vi "lab4_usrp_cp_ofdm_transceiver.vi"() -> ()   [LabVIEW 2014]
uses:
  <vilib>/addons/Modulation/Digital/General/MT Generate Bits (Galois, PN Order).vi
  <vilib>/Analysis/2dsp.llb/Inverse Complex FFT.vi
  <vilib>/Analysis/2dsp.llb/Complex FFT.vi
  <vilib>/Analysis/5stat.llb/RMS (DBL).vi
  <vilib>/addons/Modulation/Digital/Support/Common/Validators/mod_Generate Bits Validate.vi
  <vilib>/addons/Modulation/Analog/support/mod_Set Error Source.vi
  var_stop.vi
  <vilib>/addons/Modulation/Digital/Support/Common/Validators/mod_Generate Filter Coefficients Validate.vi
  <vilib>/addons/Modulation/Digital/General/subVIs/mod_Generate Filter Coefficients.vi
  <vilib>/addons/Modulation/Digital/General/subVIs/mod_Generate Bits PN Sequence.vi
  <vilib>/addons/Modulation/Digital/General/MT Generate QAM System Parameters(M).vi
  <vilib>/addons/Modulation/Digital/General/MT Apply Pulse Shaping Filter (Generic).vi
  <instrlib>/niUSRP/niUSRP Write Tx Data (CDB Cluster).vi
  <vilib>/addons/Modulation/Digital/General/MT Apply Matched Filter (Generic).vi
  <vilib>/addons/Modulation/Digital/General/MT Align to Ideal Symbols (Generic).vi
  <vilib>/addons/Modulation/Digital/General/MT Map QAM Symbols to Bits.vi
  <instrlib>/niUSRP/niUSRP Fetch Rx Data (CDB Cluster).vi
  <vilib>/addons/Modulation/niDMT.lvlib
  <vilib>/Analysis/NI_AALPro.lvlib
panel:
  out "Time domain ofdm signal":dbl[](graph)
  out "Frequency domain subcarrier magnitude":dbl[](graph)
  out "PAPR":dbl
  in  "M-QAM (16)":i32=16
  out "TX buffer":i32
  out "RX buffer":i32
  out "avg energy":dbl
  in  "TX on":bool=TRUE
  in  "power scale":dbl format="%#_13g"
  out "acc recieved bits":i32
  out "acc error bits":i32
  out "Packet number":u8
  out "Packet bytes":u32
  out "past 20 error bits":i32[](array[numeric])
  in  "min_len":i32=200
  in  "Threshold":dbl=-61.0 format="%#_13g"
  out "Accumulated BER":dbl
  out "found packet":bool
  in  "total bits (128)":i32=1600 caption="bits per packet"
  in  "message carriers":i32=120
  out "RX  constellation map":cdb[](graph)
  in  "pilot carrier":i32=32
  in  "cyclic length":i32=64
  in  "FFT size":i32=256
  in  "filter length (symbols)":i32=8
  in  "filter parameter":dbl=0.35 format="%.2f"
  in  "samples per symbol (16)":i32=4
  in  "pulse shaping filter (none)":T1(ring)=enum."Root Raised Cos"
  in  "stop":bool
  in  "number of samples":i64=20000
  out "coerced carrier frequency":dbl format="%#_6p"
  out "coerced IQ rate":dbl format="%#_6p"
  in  "Clocking and Synchronization:Reference Frequency Source":string(combo)="Internal"
  in  "RX gain":dbl format="%#_6f"
  in  "TX gain":dbl format="%#_6f"
  in  "carrier frequency":dbl=915000000.0 format="%#_6p"
  in  "IQ rate":dbl=2000000.0 format="%#_6p"
  in  "RX device names":refnum<k15>="192.168.10.3"
  in  "TX device names":refnum<k15>="192.168.10.3"
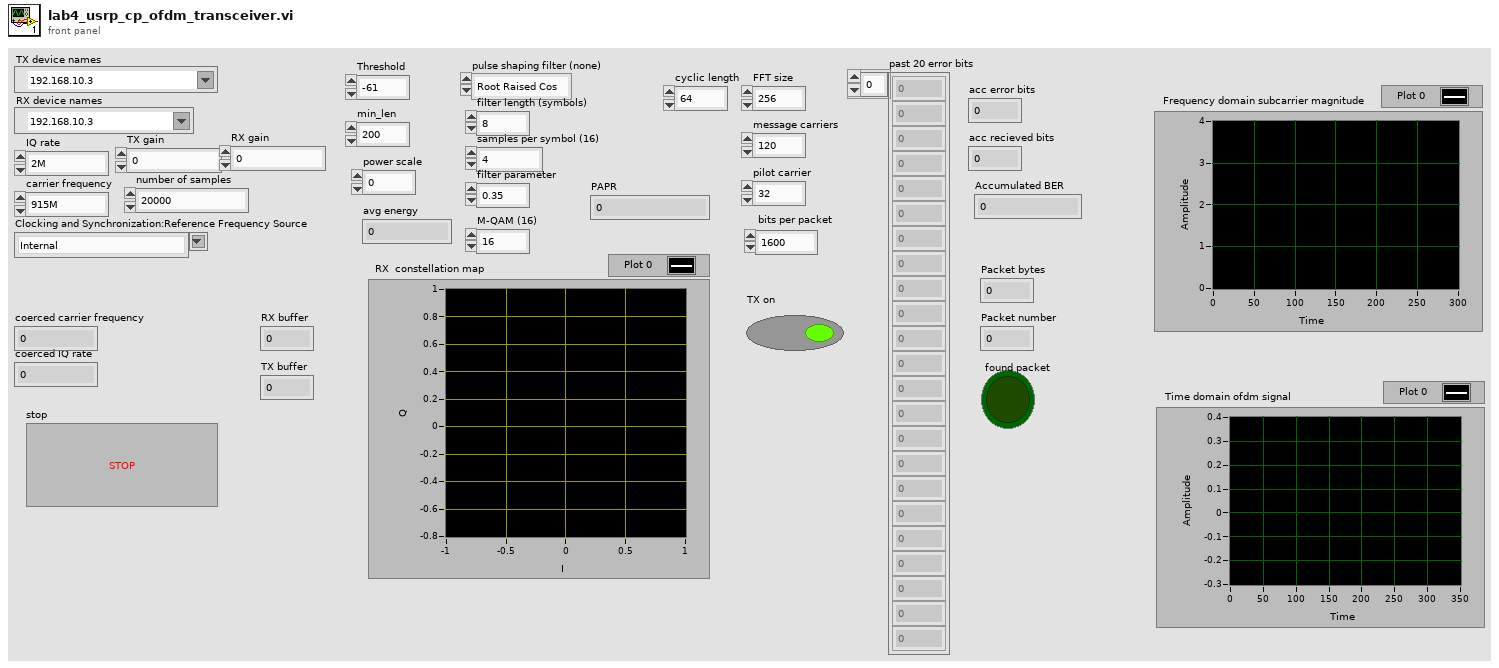
[diagram p1: front panel]
types:
  T1 = enum16{"none", "Raised Cosine", "Root Raised Cos", "Gaussian"}
  T2 = enum16{"FSK", "PSK", "QAM", "MSK", "PAM", "ASK", "CPM"}
  T3 = cluster{"samples per symbol (16)":i32, "symbol map":cdb[]}
  T4 = typedef "niAMT.lvlib/Complex Data Waveform.ctl" = cluster{"t0":dbl, "dt":dbl, "Y":cdb[]}
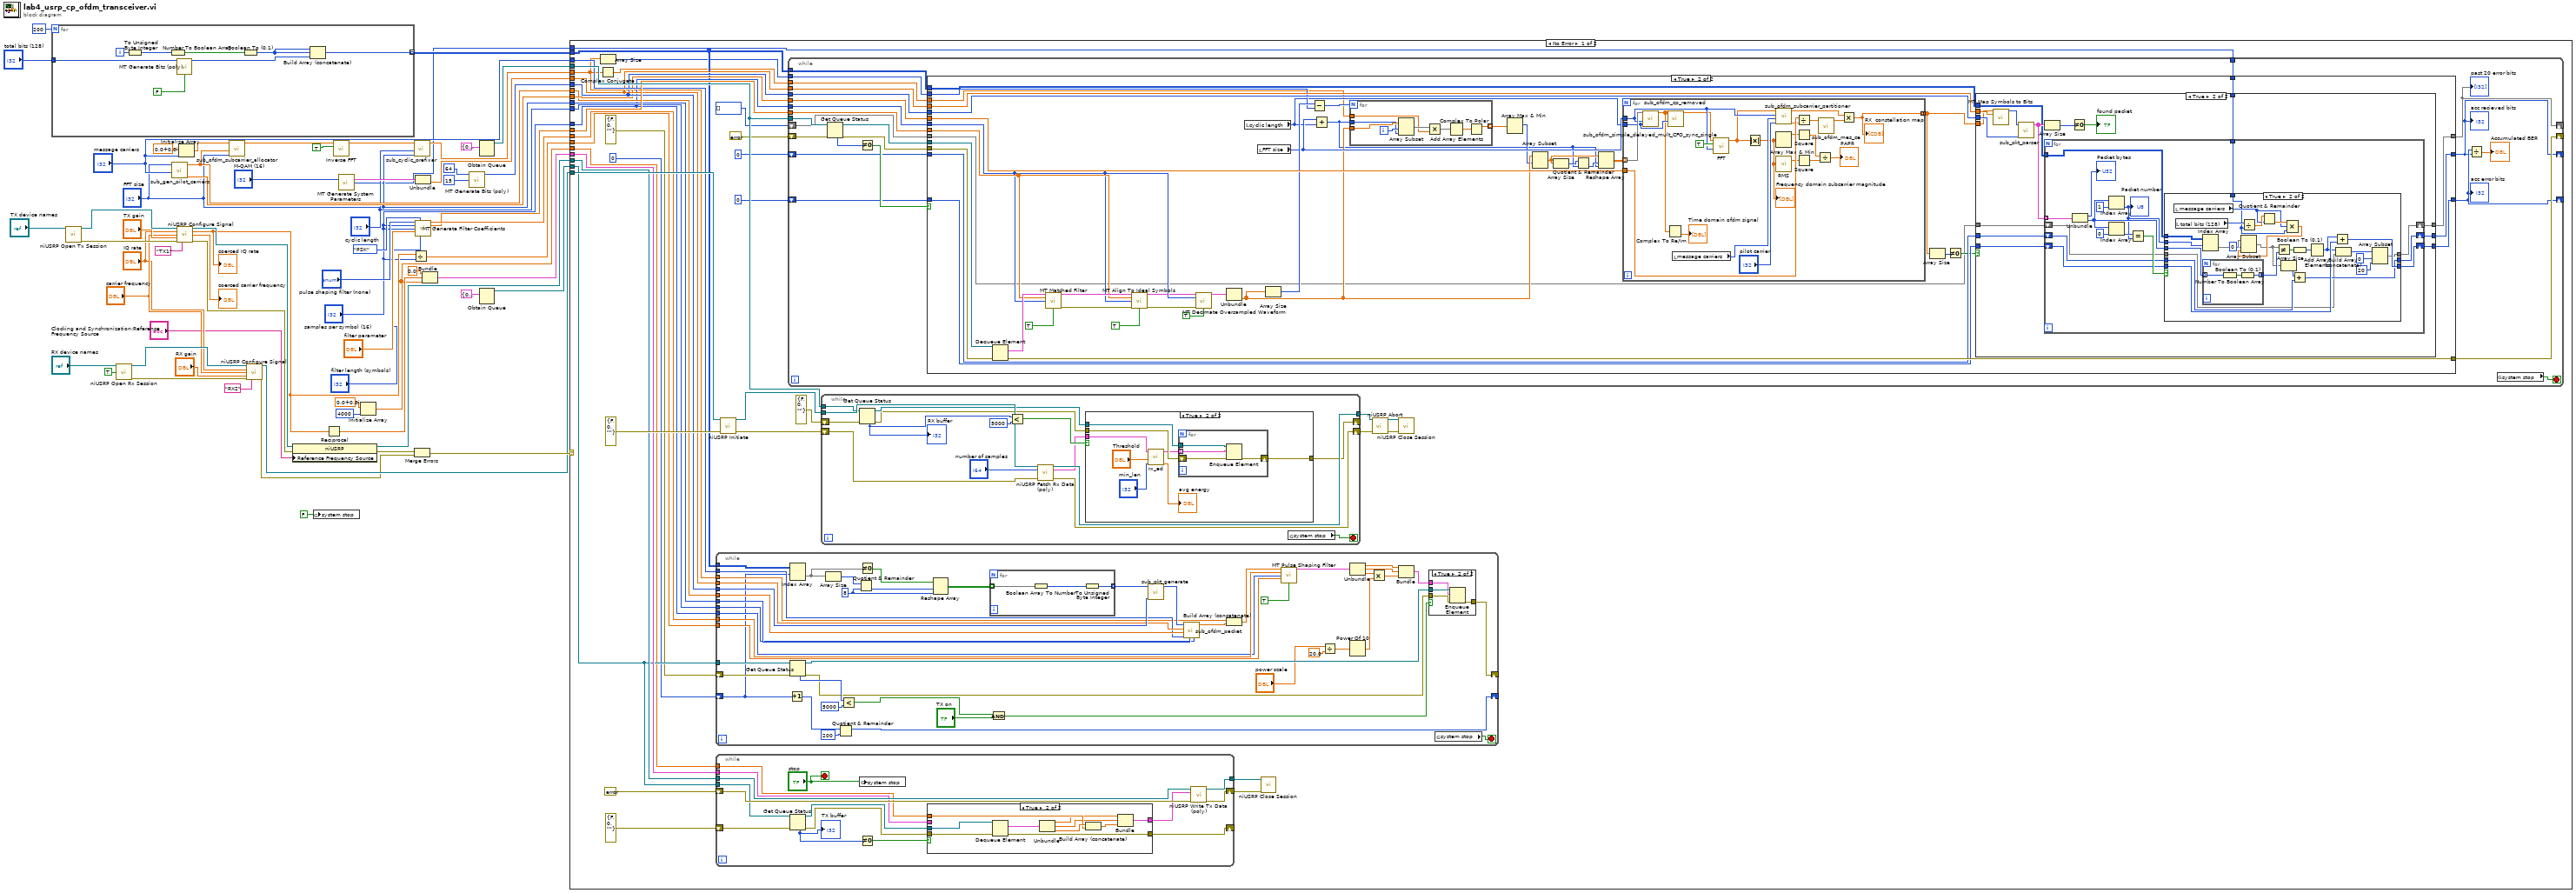
[diagram p0: block diagram]
diagram:
  n1 = for {
    N: 200 ("y") -> [_]
    tunnel: "total bits (128)" -> [w71]
    tunnel: [w64] -> w7 mode=indexing
    i -> [w69]
    n2 = To Unsigned Byte Integer(number=w69) -> (unsigned 8bit integer=w68:u8)
    n3 = Number To Boolean Array(number=w68) -> (Boolean array=w67:bool[])
    n4 = call-poly <vilib>:"MT Generate Bits (poly).vi"("total bits (128)"=w71, "reset? (T)"=FALSE) -> ("output bit stream"=w65:i8[])  [unwired: 11 in, 2 out]
    n5 = Boolean To (0,1)(Boolean=w67) -> (0, 1=w66:i16[])
    n6 = Build Array (concatenate)(w66, w66, w65) -> (w64:i16[])
  }
  n7 = call <instrlib>:"niUSRP Open Tx Session.vi"("device names"="TX device names") -> ("session handle out"=w63:refnum<k15>, "error out"=w62:errorcluster)  [unwired: 13 in]
  n8 = call <instrlib>:"niUSRP Open Rx Session.vi"("device names"="RX device names", "reset"=TRUE) -> ("session handle out"=w59:refnum<k15>, "error out"=w58:errorcluster)  [unwired: 12 in]
  n9 = call "sub_gen_pilot_carriers.vi"("message carrier"="message carriers", "FFT size"="FFT size") -> ("RX pilot carriers"=w20:cdb[], "TX pilot carriers"=w16:cdb[])  [unwired: 8 in]
  n10 = call <instrlib>:"niUSRP Configure Signal.vi"("session handle"=w63, "IQ rate"="IQ rate", "carrier frequency"="carrier frequency", "gain"="TX gain", "error in (no error)"=w62, "active antenna"="TX1") -> ("session handle out"=w30:refnum<k15>, "coerced IQ rate"=w19:dbl, "coerced carrier frequency"=→"coerced carrier frequency":dbl, "error out"=w29:errorcluster)  [unwired: 5 in, 1 out]
  "coerced IQ rate" <- w19
  n11 = Initialize Array(cdb 0.0+0.0i, "message carriers") -> (w22:cdb[])
  n12 = call "sub_ofdm_subcarrier_allocator.vi"("fft size"="FFT size", "pilot symbol"=w16, "message symbol"=w22) -> ("OFDM symbol"=w15:cdb[])  [unwired: 8 in]
  n13 = call <instrlib>:"niUSRP Configure Signal.vi"("session handle"=w59, "IQ rate"="IQ rate", "carrier frequency"="carrier frequency", "gain"="RX gain", "error in (no error)"=w58, "active antenna"="RX2") -> ("session handle out"=w2:refnum<k15>, "error out"=w1:errorcluster)  [unwired: 5 in, 3 out]
  n14 = property class="niUSRP"(reference=w30, error in=w29, "Reference Frequency Source"="Clocking and Synchronization:Reference Frequency Source") -> (reference out=w44:refnum<k15>, error out=w49:errorcluster)
  n15 = global write "var_stop.vi" "system stop"(FALSE) -> ()
  n16 = Reciprocal(x=w19) -> (1/x=w39:dbl)
  n17 = call-poly <vilib>:"Inverse FFT.vi"("shift?"=TRUE, "FFT {X}"=w15) -> ("X"=w13:cdb[])  [unwired: 8 in, 1 out]
  n18 = call-poly <vilib>:"MT Generate System Parameters.vi"("M-QAM (16)"="M-QAM (16)") -> ("QAM system parameters"=w28:T3, "bits per symbol"=w4:i32)  [unwired: 12 in, 1 out]
  n19 = Initialize Array(cdb 0.0+0.0i, 4000 ("dimension size")) -> (w6:cdb[])
  n20 = Divide(x=w19, y="samples per symbol (16)") -> (x/y=w18:dbl)
  n21 = call "sub_cyclic_prefixer.vi"("FFT size"="FFT size", "CP length"="cyclic length", "time_samples"=w13) -> ("cp ofdm symbol"=w10:cdb[])  [unwired: 8 in]
  n22 = Merge Errors(w49, w1) -> (w48:errorcluster)
  n23 = Unbundle(w28) -> ("symbol map"=w27:cdb[])  [unwired: 1 out]
  n24 = call <vilib>:"MT Generate Filter Coefficients.vi"("pulse shaping filter (none)"="pulse shaping filter (none)", "modulation type"=T2."PSK", "pulse shaping samples per symbol (16)"="samples per symbol (16)", "matched samples per symbol (16)"="samples per symbol (16)", "filter parameter"="filter parameter", "filter length (symbols)"="filter length (symbols)") -> ("pulse shaping filter coefficients"=w33:dbl[], "matched filter coefficients"=w32:dbl[])  [unwired: 7 in, 1 out]
  n25 = Bundle(0.0, w39, w6) -> (w37:cluster{dbl, dbl, cdb[]})  [unwired: 1 in]
  n26 = call-poly <vilib>:"MT Generate Bits (poly).vi"("total bits (128)"=64, "PN sequence order (9)"=15) -> ("output bit stream"=w24:i8[])  [unwired: 11 in, 2 out]
  n27 = Obtain Queue(element data type=cluster{"t0":dbl, "dt":dbl, "Y":cdb[]} {"t0"=0.0, "dt"=0.0, "Y"=[]} ("data")) -> (queue out=w45:refnum<queue>)  [unwired: 4 in, 2 out]
  n28 = Obtain Queue(element data type=cluster{"t0":dbl, "dt":dbl, "Y":cdb[]} {"t0"=0.0, "dt"=0.0, "Y"=[]} ("data")) -> (queue out=w42:refnum<queue>)  [unwired: 4 in, 2 out]
  n29 = case shown="No Error" w48 {
    tunnel: w2 -> [w109 _]
    tunnel: w45 -> [w104 _]
    tunnel: w44 -> [w99 _]
    tunnel: w42 -> [w96 _]
    tunnel: w37 -> [w97 _]
    tunnel: w33 -> [w94 _]
    tunnel: w32 -> [w93 _]
    tunnel: "message carriers" -> [w90 _]
    tunnel: "FFT size" -> [w89 _]
    tunnel: w27 -> [w88 _]
    tunnel: w24 -> [w87 _]
    tunnel: w20 -> [w86 _]
    tunnel: w18 -> [w85 _]
    tunnel: "samples per symbol (16)" -> [w82 _]
    tunnel: w16 -> [w84 _]
    tunnel: "cyclic length" -> [w83 _]
    tunnel: w10 -> [w76 _]
    tunnel: w7 -> [w80 _]
    tunnel: w6 -> [w77 _]
    tunnel: w4 -> [w72 _]
    frame No Error {
      n30 = Complex Conjugate(1:w76) -> (0:w74:cdb[])
      n31 = Array Size(array=w76) -> (size(s)=w75:i32)
      n32 = while {
        tunnel: w96 -> [w151]
        shift-right: [w153] -> _
        shift-left: errorcluster {"status"=FALSE, "code"=0, "source"=""} ("error out") -> [w152]
        tunnel: w84 -> [w143]
        tunnel: w94 -> [w150]
        tunnel: w82 -> [w149]
        tunnel: w85 -> [w148]
        tunnel: w90 -> [w142]
        tunnel: w89 -> [w141]
        tunnel: w88 -> [w144]
        tunnel: w87 -> [w146]
        tunnel: w83 -> [w140]
        tunnel: w76 -> [w139]
        tunnel: w80 -> [w136]
        shift-right: [w132] -> _
        shift-left: 0 -> [w135]
        stop <- w158 stop-if-true
        w129 = 8 ("y")
        n33 = Increment(x=w135) -> (x+1=w134:i32)
        n34 = Index Array(array=w136, index (row)=w135) -> (element=w128:i16[])  [unwired: 1 in]
        n35 = Get Queue Status(queue=w151, error in (no error)=w152) -> (queue out=w155:refnum<queue>, error out=w154:errorcluster, # elements in queue=w157:i32)  [unwired: 1 in, 5 out]
        n36 = Array Size(array=w128) -> (size(s)=w131:i32)
        n37 = Quotient & Remainder(x=w134, y=200) -> (x-y*floor(x/y)=w132:i32)  [unwired: 1 out]
        n38 = Less?(x=w157, y=5000) -> (x < y?=w114:bool)
        n39 = Quotient & Remainder(x=w131, y=w129) -> (floor(x/y)=w130:i32)  [unwired: 1 out]
        n40 = Not Equal To 0?(x=w128) -> (x != 0?=w127:bool[])
        n41 = Reshape Array(w127, w130, w129) -> (w126:bool[][])
        n42 = for {
          tunnel: w126 -> [w161] mode=indexing
          tunnel: [w159] -> w125 mode=indexing
          n43 = Boolean Array To Number(Boolean array=w161) -> (number=w160:u32)
          n44 = To Unsigned Byte Integer(number=w160) -> (unsigned 8bit integer=w159:u8)
        }
        n45 = And(x=w114, y="TX on") -> (x .and. y?=w112:bool)
        n46 = call "sub_pkt_generate.vi"("accesscode (bit)"=w146, "byte stream"=w125) -> ("bit pkt"=w145:i16[])  [unwired: 9 in]
        n47 = call "sub_ofdm_packet.vi"("CP length"=w140, "FFT size"=w141, "message carriers"=w142, "pilot symbol"=w143, "symbol map"=w144, "packet"=w145) -> ("ofdm packet"=w138:cdb[])  [unwired: 5 in]
        n48 = Build Array (concatenate)(w139, w138) -> (w137:cdb[])
        n49 = call-poly <vilib>:"MT Pulse Shaping Filter.vi"("symbols"=w137, "pulse shaping filter coefficients"=w150, "samples per symbol (16)"=w149, "symbol rate (Hz)"=w148, "reset? (T)"=TRUE) -> ("output complex waveform"=w121:T4)  [unwired: 9 in, 1 out]
        n50 = Divide(x="power scale", y=20.0) -> (x/y=w122:dbl)
        n51 = Unbundle(w121) -> ("t0"=w116:dbl, "dt"=w117:dbl, "Y"=w120:cdb[])
        n52 = Power Of 10(x=w122) -> (10^x=w119:dbl)
        n53 = Multiply(x=w120, y=w119) -> (x*y=w118:cdb[])
        n54 = Bundle("t0"=w116, "dt"=w117, w118) -> (w115:cluster{"t0":dbl, "dt":dbl, cdb[]})  [unwired: 1 in]
        n55 = case shown="True" w112 {
          tunnel: w155 -> [_ w166]
          tunnel: w154 -> [w162 w165]
          tunnel: [w162 w164] -> w153
          tunnel: w115 -> [_ w163]
          frame False {
          }
          frame True {
            n56 = Enqueue Element(queue=w166, element=w163, error in (no error)=w165) -> (error out=w164:errorcluster)  [unwired: 1 in, 2 out]
          }
        }
        n57 = global read "var_stop.vi" "system stop"() -> (w158:bool)
      }
      n58 = while {
        tunnel: [w374] -> w102
        shift-right: [w373] -> w101
        shift-left: errorcluster {"status"=FALSE, "code"=0, "source"=""} ("error out") -> [w371]
        tunnel: w99 -> [w372]
        tunnel: w96 -> [w370]
        shift-right: [w364] -> _
        shift-left: errorcluster {"status"=FALSE, "code"=0, "source"=""} ("error out") -> [w369]
        tunnel: w97 -> [w363]
        tunnel: w77 -> [w362]
        stop <- "stop" stop-if-true
        n59 = Get Queue Status(queue=w370, error in (no error)=w369) -> (queue out=w366:refnum<queue>, error out=w367:errorcluster, # elements in queue=w368:i32)  [unwired: 1 in, 5 out]
        "TX buffer" <- w368
        n60 = global write "var_stop.vi" "system stop"("stop") -> ()
        n61 = Not Equal To 0?(x=w368) -> (x != 0?=w361:bool)
        n62 = case shown="True" w361 {
          tunnel: w367 -> [w377 w386]
          tunnel: w366 -> [_ w387]
          tunnel: [w376 w378] -> w365
          tunnel: [w377 w385] -> w364
          tunnel: w363 -> [w376 _]
          tunnel: w362 -> [_ w382]
          frame False {
          }
          frame True {
            n63 = Dequeue Element(queue=w387, error in (no error)=w386) -> (element=w384:cluster{"t0":dbl, "dt":dbl, "Y":cdb[]}, error out=w385:errorcluster)  [unwired: 1 in, 2 out]
            n64 = Unbundle(w384) -> ("t0"=w379:dbl, "dt"=w380:dbl, "Y"=w383:cdb[])
            n65 = Build Array (concatenate)(w383, w382) -> (w381:cdb[])
            n66 = Bundle("t0"=w379, "dt"=w380, w381) -> (w378:cluster{"t0":dbl, "dt":dbl, cdb[]})  [unwired: 1 in]
          }
        }
        n67 = call-poly <instrlib>:"niUSRP Write Tx Data (poly).vi"("session handle"=w372, "data"=w365, "error in (no error)"=w371) -> ("session handle out"=w374:refnum<k15>, "error out"=w373:errorcluster)  [unwired: 11 in]
      }
      n68 = call <instrlib>:"niUSRP Initiate.vi"("session handle"=w109, "error in (no error)"=errorcluster {"status"=FALSE, "code"=0, "source"=""}) -> ("session handle out"=w111:refnum<k15>, "error out"=w110:errorcluster)  [unwired: 12 in]
      n69 = while {
        tunnel: w104 -> [w185]
        shift-right: [w183] -> _
        shift-left: errorcluster {"status"=FALSE, "code"=0, "source"=""} ("error out") -> [w184]
        tunnel: w93 -> [w182]
        tunnel: w82 -> [w181]
        tunnel: w86 -> [w180]
        tunnel: w88 -> [w179]
        tunnel: w87 -> [w178]
        tunnel: w80 -> [w177]
        shift-right: [w173] -> _
        shift-left: 0 -> [w175]
        shift-right: [w174] -> _
        shift-left: 0 -> [w176]
        tunnel: w75 -> [w171]
        tunnel: w74 -> [w170]
        shift-right: [w168] -> _
        shift-left: i32[] [] -> [w169]
        tunnel: w72 -> [w167]
        stop <- w190 stop-if-true
        n70 = Get Queue Status(queue=w185, error in (no error)=w184) -> (queue out=w186:refnum<queue>, error out=w187:errorcluster, # elements in queue=w189:i32)  [unwired: 1 in, 5 out]
        n71 = Not Equal To 0?(x=w189) -> (x != 0?=w188:bool)
        n72 = case shown="True" w188 {
          tunnel: w187 -> [w194 w236]
          tunnel: w186 -> [_ w235]
          tunnel: [w194 w234] -> w183
          tunnel: w182 -> [_ w226]
          tunnel: w181 -> [_ w225]
          tunnel: w180 -> [_ w229]
          tunnel: w179 -> [_ w221]
          tunnel: w178 -> [_ w220]
          tunnel: w177 -> [_ w219]
          tunnel: w176 -> [w193 w218]
          tunnel: w175 -> [w192 w217]
          tunnel: [w193 w216] -> w174
          tunnel: [w192 w215] -> w173
          tunnel: w171 -> [_ w210]
          tunnel: w170 -> [_ w206]
          tunnel: w169 -> [w191 w197]
          tunnel: [w191 w196] -> w168
          tunnel: w167 -> [_ w195]
          frame False {
          }
          frame True {
            n73 = Dequeue Element(queue=w235, error in (no error)=w236) -> (element=w233:cluster{"t0":dbl, "dt":dbl, "Y":cdb[]}, error out=w234:errorcluster)  [unwired: 1 in, 2 out]
            n74 = call-poly <vilib>:"MT Matched Filter.vi"("input complex waveform"=w233, "matched filter coefficients"=w226, "samples per symbol (16)"=w225, "reset? (T)"=TRUE) -> ("output complex waveform"=w228:T4, "error out"=w227:errorcluster)  [unwired: 10 in]
            n75 = call-poly <vilib>:"MT Align To Ideal Symbols.vi"("input complex waveform"=w228, "matched filter coefficients"=w226, "samples per symbol (16)"=w225, "error in (no error)"=w227, "reset? (T)"=TRUE) -> ("output complex waveform"=w223:T4, "error out"=w222:errorcluster)  [unwired: 8 in, 1 out]
            n76 = call <vilib>:"MT Decimate Oversampled Waveform.vi"("input complex waveform"=w223, "decimation factor"=w225, "error in (no error)"=w222, "reset? (T)"=TRUE) -> ("output complex waveform"=w231:T4)  [unwired: 10 in, 1 out]
            n77 = Unbundle(w231) -> ("Y"=w204:cdb[])  [unwired: 2 out]
            n78 = local read "cyclic length"() -> (w207:i32)
            n79 = local read "FFT size"() -> (w208:i32)
            n80 = Array Size(array=w204) -> (size(s)=w211:i32)
            n81 = Subtract(x=w211, y=w210) -> (x-y=w209:i32)
            n82 = Add(x=w208, y=w207) -> (x+y=w199:i32)
            n83 = for {
              N: w209 -> [_]
              tunnel: w204 -> [w244]
              tunnel: w199 -> [w242]
              tunnel: w206 -> [w240]
              tunnel: [w237] -> w205 mode=indexing
              i -> [w243]
              n84 = Array Subset(array=w244, index=w243, length=w242) -> (w241:cdb[])
              n85 = Multiply(x=w241, y=w240) -> (x*y=w239:cdb[])
              n86 = Add Array Elements(numeric array=w239) -> (sum=w238:cdb)
              n87 = Complex To Polar(r * e^(i*theta)=w238) -> (r=w237:dbl)  [unwired: 1 out]
            }
            n88 = Array Max & Min(array=w205) -> (max index (indices)=w203:i32)  [unwired: 3 out]
            n89 = Array Subset(array=w204, index=w203) -> (w201:cdb[])  [unwired: 1 in]
            n90 = Array Size(array=w201) -> (size(s)=w202:i32)
            n91 = Quotient & Remainder(x=w202, y=w199) -> (floor(x/y)=w200:i32)  [unwired: 1 out]
            n92 = Reshape Array(w201, w200, w199) -> (w198:cdb[][])
            n93 = for {
              tunnel: w198 -> [w323] mode=indexing
              tunnel: w207 -> [w321]
              tunnel: w208 -> [w322]
              tunnel: [w329] -> w214 mode=concatenating
              tunnel: w229 -> [w326]
              n94 = call "sub_ofdm_simple_delayed_mult_CFO_sync_single.vi"("CP length"=w321, "FFT size"=w322, "time samples"=w323) -> ("sync ofdm symbol"=w311:cdb[])  [unwired: 8 in]
              n95 = call "sub_ofdm_cp_removed.vi"("CP length"=w321, "time ofdm symbol"=w311) -> ("cp removed ofdm symbol"=w313:cdb[])  [unwired: 9 in]
              n96 = Complex To Re/Im(x + iy=w311) -> (y=→"Time domain ofdm signal":dbl[])  [unwired: 1 out]
              n97 = local read "message carriers"() -> (w328:i32)
              n98 = call-poly <vilib>:"FFT.vi"("FFT size"=w322, "shift?"=TRUE, "X"=w313) -> ("FFT {X}"=w320:cdb[])  [unwired: 7 in, 1 out]
              n99 = Absolute Value(x=w320) -> (abs(x)=w314:dbl[])
              "Frequency domain subcarrier magnitude" <- w314
              n100 = call "sub_ofdm_subcarrier_partitioner.vi"("pilot carrier"="pilot carrier", "message carrier"=w328, "FFT size"=w322, "received symbol"=w320) -> ("pilot subcarriers"=w325:cdb[], "message subcarriers"=w327:cdb[])  [unwired: 6 in]
              n101 = Array Max & Min(array=w314) -> (max value=w319:dbl)  [unwired: 3 out]
              n102 = call-poly <vilib>:"RMS.vi"("X"=w314) -> ("rms value"=w317:dbl)  [unwired: 1 out]
              n103 = Divide(x=w326, y=w325) -> (x/y=w324:cdb[])
              n104 = Square(x=w319) -> (x^2=w318:dbl)
              n105 = Square(x=w317) -> (x^2=w316:dbl)
              n106 = Divide(x=w318, y=w316) -> (x/y=→"PAPR":dbl)
              n107 = call "sub_ofdm_mes_ce.vi"("ZF channel estimates"=w324) -> ("interpolated mes carrier CE"=w330:cdb[])  [unwired: 10 in]
              n108 = Multiply(x=w327, y=w330) -> (x*y=w329:cdb[])
              "RX  constellation map" <- w329
            }
            n109 = Array Size(array=w214) -> (size(s)=w213:i32)
            n110 = Not Equal To 0?(x=w213) -> (x != 0?=w212:bool)
            n111 = case shown="True" w212 {
              tunnel: w221 -> [_ w262]
              tunnel: w220 -> [_ w260]
              tunnel: w219 -> [_ w256]
              tunnel: w218 -> [w247 w255]
              tunnel: w217 -> [w246 w254]
              tunnel: [w247 w253] -> w216
              tunnel: [w246 w252] -> w215
              tunnel: w214 -> [_ w251]
              tunnel: w197 -> [w245 w250]
              tunnel: [w245 w249] -> w196
              tunnel: w195 -> [_ w248]
              frame False {
              }
              frame True {
                n112 = call-poly <vilib>:"MT Map Symbols to Bits.vi"("symbols"=w251, "symbol map"=w262) -> ("output bit stream"=w261:i8[])  [unwired: 12 in, 1 out]
                n113 = call "sub_pkt_parser.vi"("accesscode (bit)"=w260, "bitstream"=w261) -> ("parsed packet"=w257:cluster{"t":u32, "byte_array":u8[]}[])  [unwired: 9 in]
                n114 = Array Size(array=w257) -> (size(s)=w259:i32)
                n115 = for {
                  tunnel: w257 -> [w278] mode=indexing
                  tunnel: w256 -> [w272]
                  shift-right: [w269] -> w253
                  shift-left: w255 -> [w270]
                  shift-right: [w267] -> w252
                  shift-left: w254 -> [w268]
                  shift-right: [w265] -> w249
                  shift-left: w250 -> [w266]
                  tunnel: w248 -> [w263]
                  n116 = Unbundle(w278) -> ("t"=→"Packet bytes":u32, "byte_array"=w273:u8[])
                  n117 = Index Array(array=w273, index=1) -> (element=w271:u8)
                  "Packet number" <- w271
                  n118 = Index Array(array=w273, index=0) -> (element=w275:u8)
                  n119 = Equal?(x=w275, y=w271) -> (x = y?=w274:bool)
                  n120 = case shown="True" w274 {
                    tunnel: w273 -> [_ w293]
                    tunnel: w272 -> [_ w307]
                    tunnel: w271 -> [_ w306]
                    tunnel: w270 -> [w281 w303]
                    tunnel: [w281 w302] -> w269
                    tunnel: w268 -> [w280 w301]
                    tunnel: [w280 w300] -> w267
                    tunnel: w266 -> [w279 w299]
                    tunnel: [w279 w294] -> w265
                    tunnel: w263 -> [_ w288]
                    frame False {
                    }
                    frame True {
                      n121 = local read "message carriers"() -> (w289:i32)
                      n122 = local read "total bits (128)"() -> (w292:i32)
                      n123 = Index Array(array=w307, index (row)=w306) -> (element=w287:i16[])  [unwired: 1 in]
                      n124 = for {
                        tunnel: w293 -> [w310] mode=indexing
                        tunnel: [w308] -> w284 mode=concatenating
                        n125 = Number To Boolean Array(number=w310) -> (Boolean array=w309:bool[])
                        n126 = Boolean To (0,1)(Boolean=w309) -> (0, 1=w308:i16[])
                      }
                      n127 = Divide(x=w292, y=w288) -> (x/y=w291:dbl)
                      n128 = Quotient & Remainder(x=w291, y=w289) -> (floor(x/y)=w290:dbl)  [unwired: 1 out]
                      n129 = Compound Arithmetic op=MULTIPLY(w290, w289, w288) -> (w285:dbl)
                      n130 = Array Subset(array=w287, index=0, length=w285) -> (w283:i16[])
                      n131 = Not Equal?(x=w283, y=w284) -> (x != y?=w305:bool[])
                      n132 = Array Size(array=w283) -> (size(s)=w282:i32)
                      n133 = Boolean To (0,1)(Boolean=w305) -> (0, 1=w304:i16[])
                      n134 = Add(x=w282, y=w301) -> (x+y=w300:i32)
                      n135 = Add Array Elements(numeric array=w304) -> (sum=w298:i16)
                      n136 = Add(x=w298, y=w303) -> (x+y=w302:i32)
                      n137 = Build Array (concatenate)(w298, w299) -> (w297:i32[])
                      n138 = Array Subset(array=w297, index=0, length=20) -> (w294:i32[])
                    }
                  }
                }
                n139 = Not Equal To 0?(x=w259) -> (x != 0?=→"found packet":bool)
              }
            }
          }
        }
        "past 20 error bits" <- w168
        "acc error bits" <- w174
        "acc recieved bits" <- w173
        n140 = Divide(x=w174, y=w173) -> (x/y=→"Accumulated BER":dbl)
        n141 = global read "var_stop.vi" "system stop"() -> (w190:bool)
      }
      n142 = while {
        tunnel: w111 -> [w347]
        shift-right: [w340] -> w106
        shift-left: w110 -> [w346]
        tunnel: [w341] -> w107
        tunnel: w104 -> [w337]
        shift-right: [w335] -> _
        shift-left: errorcluster {"status"=FALSE, "code"=0, "source"=""} ("error out") -> [w334]
        stop <- w333 stop-if-true
        n143 = Get Queue Status(queue=w337, error in (no error)=w334) -> (queue out=w338:refnum<queue>, error out=w336:errorcluster, # elements in queue=w344:i32)  [unwired: 1 in, 5 out]
        "RX buffer" <- w344
        n144 = Less?(x=w344, y=5000) -> (x < y?=w342:bool)
        n145 = call-poly <instrlib>:"niUSRP Fetch Rx Data (poly).vi"("session handle"=w347, "number of samples"="number of samples", "error in (no error)"=w346) -> ("session handle out"=w341:refnum<k15>, "data"=w339:cluster{"t0":dbl, "dt":dbl, "Y":cdb[]}, "error out"=w340:errorcluster)  [unwired: 9 in, 1 out]
        n146 = case shown="True" w342 {
          tunnel: w339 -> [_ w353]
          tunnel: w338 -> [_ w354]
          tunnel: w336 -> [w348 w356]
          tunnel: [w348 w355] -> w335
          frame False {
          }
          frame True {
            n147 = call "rx_ed.vi"("min_len"="min_len", "Threshold"="Threshold", "Wavefrom"=w353) -> ("avg energy"=→"avg energy":dbl, "extract wav"=w350:cluster{"t0":dbl, "dt":dbl, cdb[]}[])  [unwired: 7 in]
            n148 = for {
              tunnel: w354 -> [w358]
              shift-right: [w359] -> w355
              shift-left: w356 -> [w360]
              tunnel: w350 -> [w357] mode=indexing
              n149 = Enqueue Element(queue=w358, element=w357, error in (no error)=w360) -> (error out=w359:errorcluster)  [unwired: 1 in, 2 out]
            }
          }
        }
        n150 = global read "var_stop.vi" "system stop"() -> (w333:bool)
      }
      n151 = call <instrlib>:"niUSRP Close Session.vi"("session handle"=w102, "error in (no error)"=w101) -> ()  [unwired: 13 in, 1 out]
      n152 = call <instrlib>:"niUSRP Abort.vi"("session handle"=w107, "error in (no error)"=w106) -> ("session handle out"=w92:refnum<k15>, "error out"=w91:errorcluster)  [unwired: 12 in]
      n153 = call <instrlib>:"niUSRP Close Session.vi"("session handle"=w92, "error in (no error)"=w91) -> ()  [unwired: 13 in, 1 out]
    }
    frame Error {
    }
  }
